vi "Robot Drive Manual - Arcade.vi"(0 "Gear Shift Data":T1, 1 "Rotation Multiplier":dbl, 2 "Right Side Bias":dbl, 3 "Left Side Bias":dbl, 5 "High Gear Multiplier":dbl, 7 "X Axis value":dbl, 9 "Low Gear Multiplier":dbl, 11 "Y Axis value":dbl, 12 "RobotDriveDevRef":T2, 13 "Gear Shift Throttle Limit":dbl) -> (4 "Motor Values":dbl[](array[numeric]))   [LabVIEW 2016]
uses:
  <vilib>/Rock Robotics/WPI/RobotDrive/WPI_RobotDriveDevRef.ctl
  <vilib>/Rock Robotics/WPI/MotorControl/WPI_MotorControlDeviceRef.ctl
  <vilib>/Rock Robotics/WPI/MotorControl/WPI_MotorControlType.ctl
  <vilib>/Rock Robotics/SystemInterfaces/DIO/FPGA_DIOPWMChannel.ctl
  <vilib>/Rock Robotics/WPI/PWM/WPI_PWMDeadband.ctl
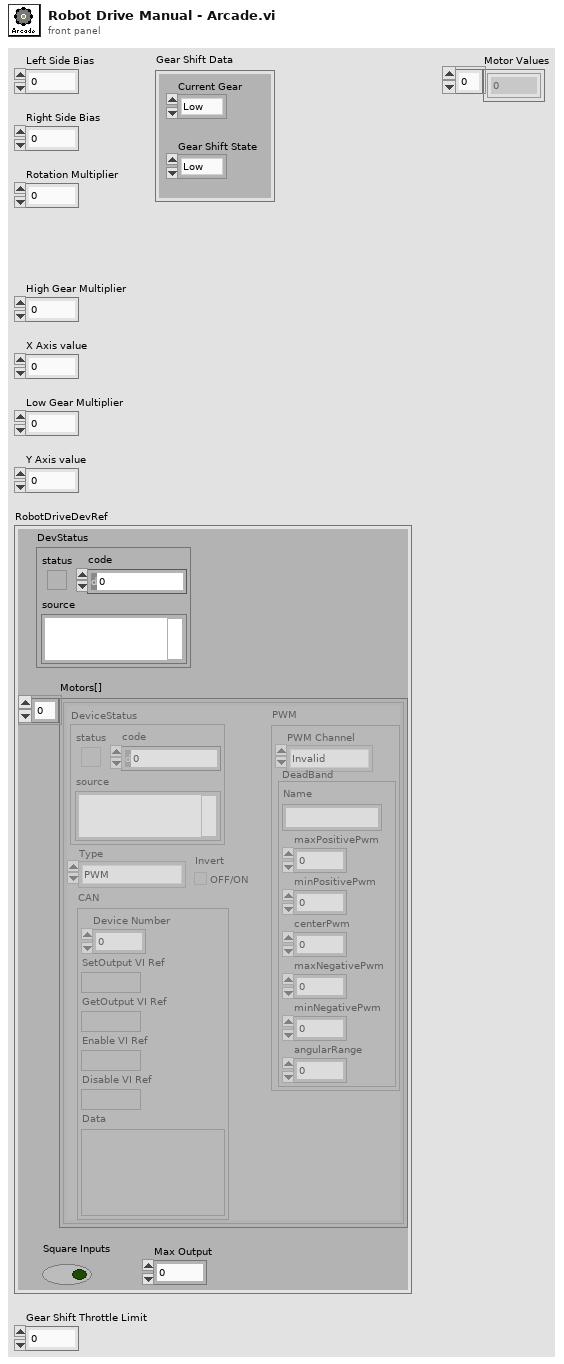
[diagram p1: front panel]
types:
  T1 = cluster{"Current Gear":enum16{"Low", "High"}, "Gear Shift State":enum16{"Low", "Shifting", "High"}}
  T2 = typedef "WPI_RobotDriveDevRef.ctl" = cluster{"DevStatus":errorcluster, "Motors[]":T3[], "Square Inputs":bool, "Max Output":dbl}
  T3 = typedef "WPI_MotorControlDeviceRef.ctl" = cluster{"DeviceStatus":errorcluster, "Type":T4, "PWM":cluster{"PWM Channel":T5, "DeadBand":T6}, "CAN":cluster{"Device Number":u8, "SetOutput VI Ref":variant, "GetOutput VI Ref":variant, "Enable VI Ref":variant, "Disable VI Ref":variant, "Data":variant}, "Invert":bool}
  T4 = typedef "WPI_MotorControlType.ctl" = enum16{"PWM", "CAN"}
  T5 = typedef "FPGA_DIOPWMChannel.ctl" = enum8{"PWM 0", "PWM 1", "PWM 2", "PWM 3", "PWM 4", "PWM 5", "PWM 6", "PWM 7", "PWM 8", "PWM 9", "PWM MXP 0", "PWM MXP 1", "PWM MXP 2", "PWM MXP 3", "PWM MXP 4", "PWM MXP 5", "PWM MXP 6", "PWM MXP 7", "PWM MXP 8", "PWM MXP 9", "Invalid"}
  T6 = typedef "WPI_PWMDeadband.ctl" = cluster{"Name":string, "maxPositivePwm":i32, "minPositivePwm":i32, "centerPwm":i32, "maxNegativePwm":i32, "minNegativePwm":i32, "angularRange":u16}
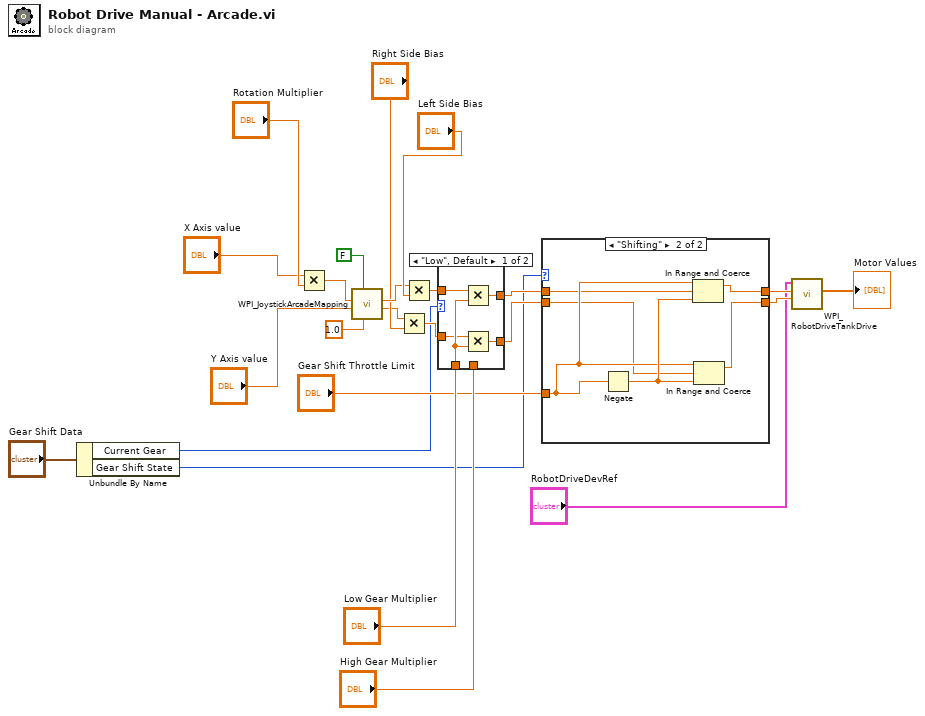
[diagram p0: block diagram]
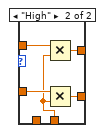
[diagram p2: hidden frame]
diagram:
  n1 = Unbundle By Name("Gear Shift Data") -> ("Current Gear"=w2:enum16{"Low", "High"}, "Gear Shift State"=w1:enum16{"Low", "Shifting", "High"})
  n2 = Multiply(x="X Axis value", y="Rotation Multiplier") -> (x*y=w19:dbl)
  n3 = call <vilib>:"WPI_JoystickArcadeMapping.vi"("Max Output"=1.0, "Square Inputs"=FALSE, "Y axis value"="Y Axis value", "X axis value"=w19) -> ("Right Motor Value"=w9:dbl, "Left Motor Value"=w13:dbl)  [unwired: 6 in]
  n4 = Multiply(x=w9, y="Right Side Bias") -> (x*y=w16:dbl)
  n5 = Multiply(x=w13, y="Left Side Bias") -> (x*y=w15:dbl)
  n6 = case shown="\"Low\", Default" w2 {
    tunnel: w15 -> [w28 w34]
    tunnel: w16 -> [w27 w33]
    tunnel: [w25 w32] -> w22
    tunnel: [w26 w31] -> w21
    tunnel: "Low Gear Multiplier" -> [w29 _]
    tunnel: "High Gear Multiplier" -> [_ w30]
    frame "Low", Default {
      n7 = Multiply(x=w28, y=w29) -> (x*y=w26:dbl)
      n8 = Multiply(x=w27, y=w29) -> (x*y=w25:dbl)
    }
    frame "High" {
      n9 = Multiply(x=w34, y=w30) -> (x*y=w31:dbl)
      n10 = Multiply(x=w33, y=w30) -> (x*y=w32:dbl)
    }
  }
  n11 = case shown="\"Shifting\"" w1 {
    tunnel: [w36 w38] -> w23
    tunnel: w21 -> [w36 w40]
    tunnel: [w35 w37] -> w24
    tunnel: w22 -> [w35 w39]
    tunnel: "Gear Shift Throttle Limit" -> [_ w41]
    frame Default {
    }
    frame "Shifting" {
      n12 = Negate(x=w41) -> (-x=w42:dbl)
      n13 = In Range and Coerce(upper limit=w41, x=w40, lower limit=w42) -> (coerced(x)=w38:dbl)  [unwired: 1 out]
      n14 = In Range and Coerce(upper limit=w41, x=w39, lower limit=w42) -> (coerced(x)=w37:dbl)  [unwired: 1 out]
    }
  }
  n15 = call <vilib>:"WPI_RobotDriveTankDrive.vi"("Right axis value"=w24, "Left axis value"=w23, "RobotDriveDevRef"="RobotDriveDevRef") -> ("Motor Values"=→"Motor Values":dbl[])  [unwired: 6 in, 2 out]
